vi "Rotate LM Array.vi"(8 "error in (no error)":errorcluster, 10 "SLAM In":T1, 11 "Observed LM Array":T3(array[cluster])) -> (0 "error out":errorcluster, 2 "SLAM Out":T1, 3 "Rotated Observed LM Array":T3(array[cluster]))   [LabVIEW 2009]
uses:
  Controls/SLAM.ctl
  <vilib>/Analysis/Matrix/Datatypes/RealMatrix.ctl
  <vilib>/Analysis/baseanly.llb/Real A x B.vi
  <vilib>/Analysis/Matrix/NI_Matrix.lvlib
  <vilib>/Analysis/NI_AALBase.lvlib
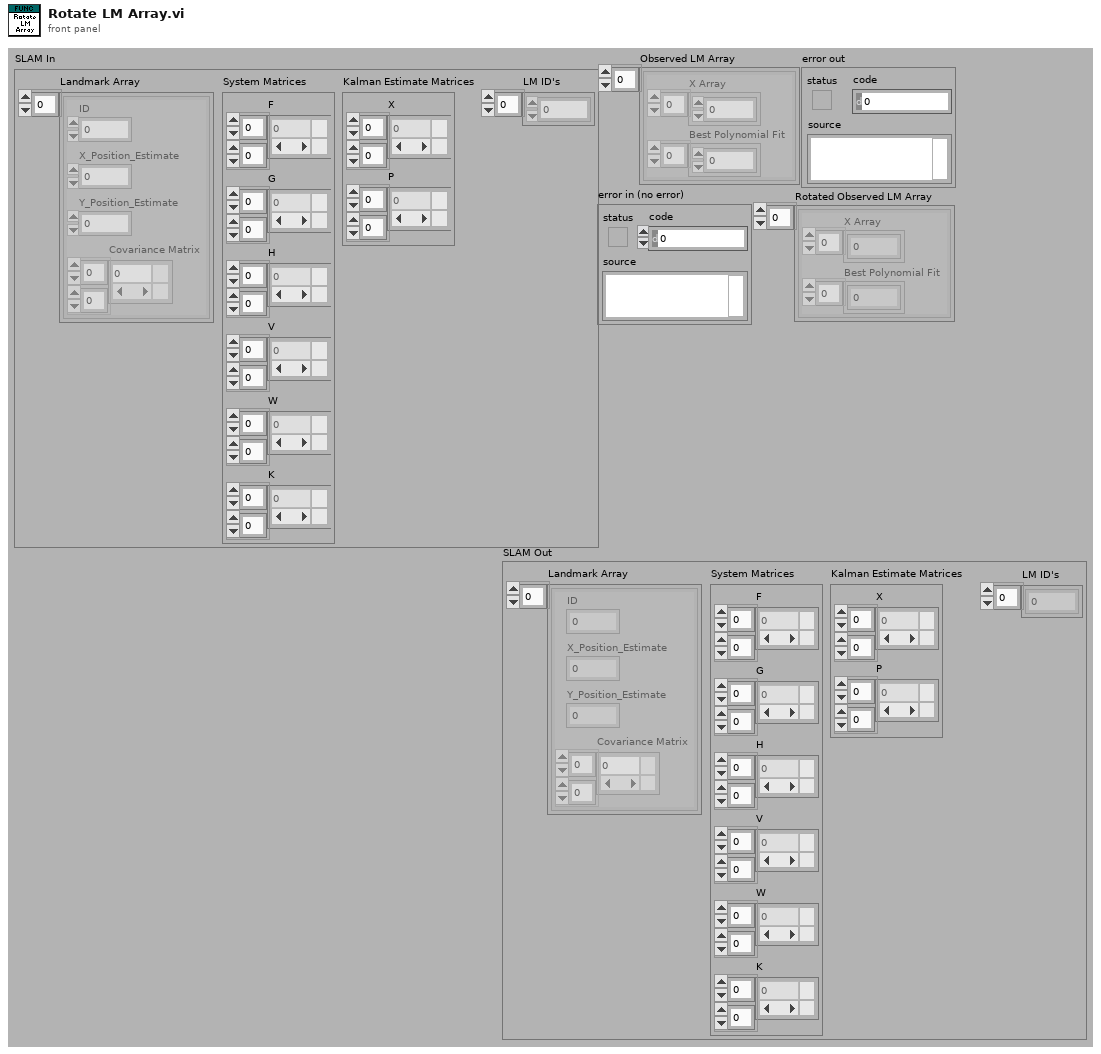
[diagram p1: front panel]
types:
  T1 = typedef "SLAM.ctl" = cluster{"Landmark Array":cluster{"ID":dbl, "X_Position_Estimate":dbl, "Y_Position_Estimate":dbl, "Covariance Matrix":T2}[], "System Matrices":cluster{"F":T2, "G":T2, "H":T2, "V":T2, "W":T2, "K":T2}, "Kalman Estimate Matrices":cluster{"X":T2, "P":T2}, "LM ID's":dbl[]}
  T2 = typedef "NI_Matrix.lvlib/RealMatrix.ctl" = dbl[][]
  T3 = cluster{"X Array":dbl[], "Best Polynomial Fit":dbl[]}[]
  T4 = cluster{"X Array":dbl[], "Best Polynomial Fit":dbl[]}
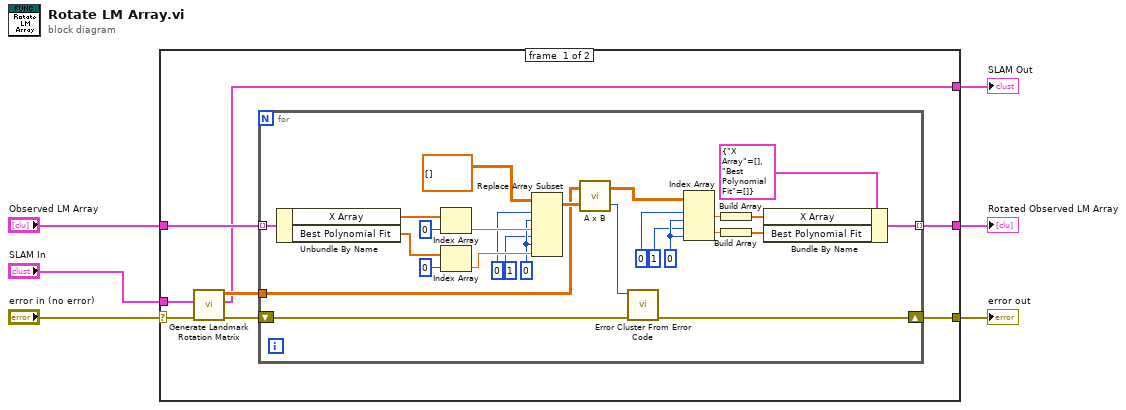
[diagram p0: block diagram]
diagram:
  n1 = case shown="No Error" "error in (no error)" {
    selector: "error in (no error)" -> [w7 w41]
    tunnel: "SLAM In" -> [w12 _]
    tunnel: "Observed LM Array" -> [w11 _]
    tunnel: [w10 w41] -> w4
    tunnel: [w9 _] -> w3
    tunnel: [w8 _] -> w2
    frame #0 {
      n2 = call "Generate Landmark Rotation Matrix.vi"("error in (no error)"=w7, "SLAM In"=w12) -> ("error out"=w13:errorcluster, "SLAM Out"=w8:T1, "Rotation matrix"=w14:T2)  [unwired: 7 in]
      n3 = for {
        shift-right: [w19] -> w10
        shift-left: w13 -> [w18]
        tunnel: w11 -> [w17] mode=indexing
        tunnel: [w21] -> w9 mode=indexing
        tunnel: w14 -> [w16]
        w40 = 0 ("index (col)")
        w34 = 0 ("index (col)")
        n4 = Unbundle By Name(w17) -> ("X Array"=w28:dbl[], "Best Polynomial Fit"=w27:dbl[])
        n5 = Index Array(array=w28, index=0) -> (element=w36:dbl)
        n6 = Index Array(array=w27, index=0) -> (element=w37:dbl)
        n7 = Replace Array Subset(array=T2 [] ("matrix"), new element #1=w36, index (row) #1=0 ("index (col)"), index (col) #1=w34, new element #2=w37, index (row) #2=1 ("index (col)"), index (col) #2=w34) -> (w31:T2)
        n8 = call-poly <vilib>:"A x B.vi"("B"=w31, "A"=w16) -> ("error"=w20:i32, "A x B"=w15:T2)
        n9 = call <vilib>:"Error Cluster From Error Code.vi"("error in (no error)"=w18, "error code (0)"=w20) -> ("error out"=w19:errorcluster)  [unwired: 7 in]
        n10 = Index Array(array=w15, index (row) #1=0 ("index (col)"), index (col) #1=w40, index (row) #2=1 ("index (col)"), index (col) #2=w40) -> (element #1=w25:dbl, element #2=w24:dbl)
        n11 = Build Array(w25) -> (w23:dbl[])
        n12 = Build Array(w24) -> (w22:dbl[])
        n13 = Bundle By Name(cluster=T4 {"X Array"=[], "Best Polynomial Fit"=[]} ("input cluster"), "X Array"=w23, "Best Polynomial Fit"=w22) -> (w21:T4)
      }
    }
    frame #1 {
    }
  }
  "error out" <- w4
  "Rotated Observed LM Array" <- w3
  "SLAM Out" <- w2
